vi "send pcan.vi"(7 "len":i32, 8 "error in (no error)":errorcluster, 9 "data":string, 10 "can_id":i32, 11 "sock":i32) -> (0 "error out":errorcluster, 1 "data out":string, 3 "function return":i32)   [LabVIEW 2024, in "libsocketcan_fd.lvlib"]
doc: "int send_pcan(int sock, int can_id, unsigned char *data, int len);"
uses:
  <userlib>/libsocketcan_fd/libsocketcan_fd.lvlib
  home/lvuser/natinst/bin/libsocketcan_fd.so
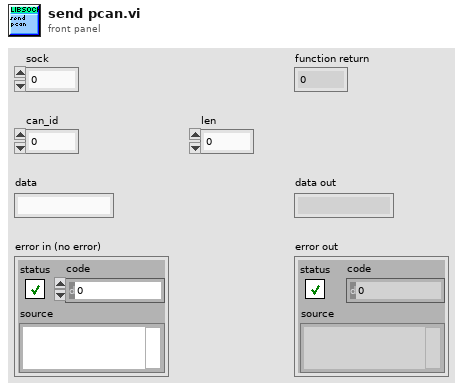
[diagram p1: front panel]
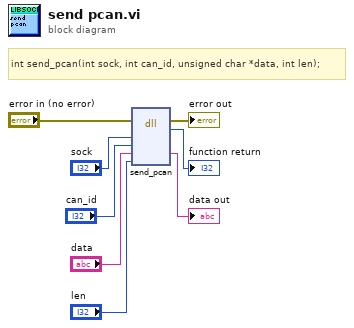
[diagram p0: block diagram]
diagram:
  # "int send_pcan(int sock, int can_id, unsigned char *data, int len);"
  n1 = dll-call lib="home/lvuser/natinst/bin/libsocketcan_fd.so" fn="send_pcan"(error in="error in (no error)", "sock"="sock", "can_id"="can_id", "data"="data", "len"="len") -> (error out=→"error out":errorcluster, "return type"=→"function return":i32, "data"=→"data out":string)  [unwired: 5 in, 1 out]
